vi "Constructor_JQMHStartup.vi"(7 "Autoshutdown? (T)":bool, 8 "error in (no error)":errorcluster, 10 "StartupParams":variant, 11 "Already Running?":bool) -> (0 "error out":errorcluster, 3 "JQMHStartup out":refnum<class "RQMHStartup.lvclass">)   [LabVIEW 2024, in "RQMHStartup.lvclass"]
uses:
  RQMHStartup.lvclass
  Shared/Died.ctl
  Message.ctl
  Command.ctl
  RQMHStartup.lvclass/RQMHStartup.ctl
  Shared/JQMHShared.lvlib
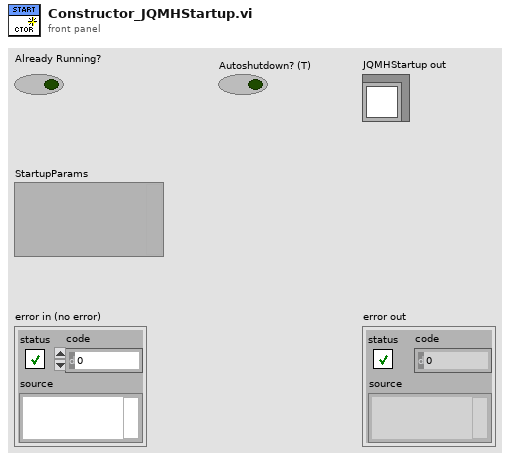
[diagram p1: front panel]
types:
  T1 = typedef "RQMHStartup.lvclass/Message.ctl" = cluster{"Command":T2, "Data":variant}
  T2 = typedef "RQMHStartup.lvclass/Command.ctl" = enum16{"Default", "No Override", "Error", "ACK Created", "ACK Mod Reg", "ACK Caller Reg"}
  T3 = typedef "JQMHShared.lvlib/Died.ctl" = bool
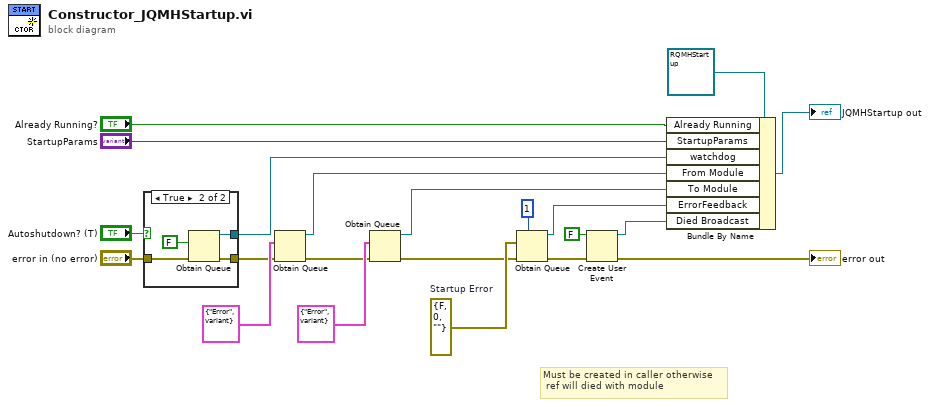
[diagram p0: block diagram]
diagram:
  w10 = errorcluster {"status"=FALSE, "code"=0, "source"=""}  # Startup Error
  # "Must be created in caller otherwise\n ref will died with module"
  n1 = case shown="True" "Autoshutdown? (T)" {
    tunnel: [_ w25] -> w6
    tunnel: "error in (no error)" -> [w22 w24]
    tunnel: [w22 w23] -> w15
    frame False {
    }
    frame True {
      n2 = Obtain Queue(element data type=FALSE, error in (no error)=w24) -> (queue out=w25:refnum<queue>, error out=w23:errorcluster)  [unwired: 3 in, 1 out]
    }
  }
  n3 = Obtain Queue(element data type=T1 {"Command"=enum."Error", "Data"=variant} ("Handshake"), error in (no error)=w15) -> (queue out=w7:refnum<queue>, error out=w4:errorcluster)  [unwired: 3 in, 1 out]
  n4 = Obtain Queue(element data type=T1 {"Command"=enum."Error", "Data"=variant} ("Handshake"), error in (no error)=w4) -> (queue out=w2:refnum<queue>, error out=w3:errorcluster)  [unwired: 3 in, 1 out]
  n5 = Obtain Queue(max queue size (-1, unlimited)=1, element data type=w10, error in (no error)=w3) -> (queue out=w9:refnum<queue>, error out=w11:errorcluster)  [unwired: 2 in, 1 out]
  n6 = Create User Event(user event datatype=T3 FALSE ("Died"), error in=w11) -> (user event=w14:refnum<user-event>, error out=→"error out":errorcluster)
  n7 = Bundle By Name(cluster=refnum<class "RQMHStartup.lvclass"> refnum ("JQMHStartup in"), "Already Running"="Already Running?", "StartupParams"="StartupParams", "watchdog"=w6, "From Module"=w7, "To Module"=w2, "ErrorFeedback"=w9, "Died Broadcast"=w14) -> (→"JQMHStartup out":refnum<class "RQMHStartup.lvclass">)
